vi "Cal BC (VIRef).vi"(8 "error in (no error)":errorcluster, 10 "BC in":variant, 11 "Domain_Evolut_1D in":refnum<class "NI_Domain_Evolut_1D.lvclass">) -> (0 "error out":errorcluster, 2 "BC out":variant, 3 "Domain_Evolut_1D out":refnum<class "NI_Domain_Evolut_1D.lvclass">)   [LabVIEW 2017, in "NI_PDE.lvlib" / "NI_Domain_Evolut_1D.lvclass"]
uses:
  <vilib>/gmath/pde.llb/DomainClass/Domain_Evolut_1D/NI_Domain_Evolut_1D.lvclass
  <vilib>/gmath/pde.llb/BCClass/BC_Evolut_1D_Numeric/BC Data.ctl
  <vilib>/gmath/pde.llb/Common/PDE_BC Type.ctl
  <vilib>/gmath/pde.llb/Common/PDE_BC Position 1D.ctl
  <vilib>/gmath/pde.llb/BCClass/BC_Evolut_1D_VIRef/BC Data.ctl
  <vilib>/gmath/pde.llb/DomainClass/Domain_Evolut_1D/NI_Domain_Evolut_1D.lvclass/NI_Domain_Evolut_1D.ctl
  <vilib>/Analysis/1siggen.llb/Ramp Pattern by Samples.vi
  <vilib>/gmath/NI_PDE.lvlib
  <vilib>/gmath/pde.llb/BCClass/BC_Evolut_1D_Numeric/NI_BC_Evolut_1D_Numeric.lvclass
  <vilib>/gmath/pde.llb/BCClass/BC_Evolut_1D_VIRef/NI_BC_Evolut_1D_VIRef.lvclass
  <vilib>/Analysis/NI_AALBase.lvlib
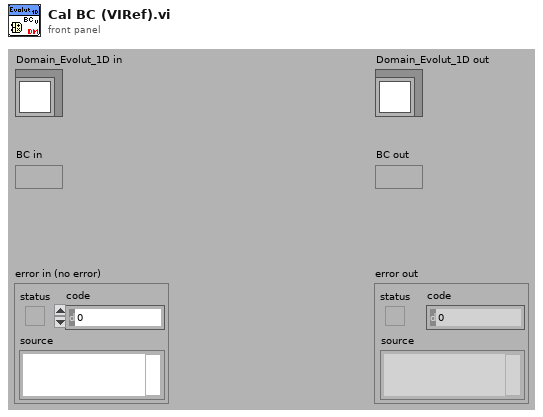
[diagram p1: front panel]
types:
  T1 = typedef "NI_PDE.lvlib/NI_BC_Evolut_1D_VIRef.lvclass/BC Data.ctl" = cluster{"type":T2, "position":T3, "G":refnum<vi>, "data":variant}
  T2 = typedef "NI_PDE.lvlib/PDE_BC Type.ctl" = i32
  T3 = typedef "NI_PDE.lvlib/PDE_BC Position 1D.ctl" = i32
  T4 = typedef "NI_PDE.lvlib/NI_BC_Evolut_1D_Numeric.lvclass/BC Data.ctl" = cluster{"type":T2, "position":T3, "G":dbl[]}
  T5 = cluster{"initial t":dbl, "final t":dbl, "# of t-points":i32}
  T6 = cluster{"start x":dbl, "end x":dbl, "# of x-points":i32}
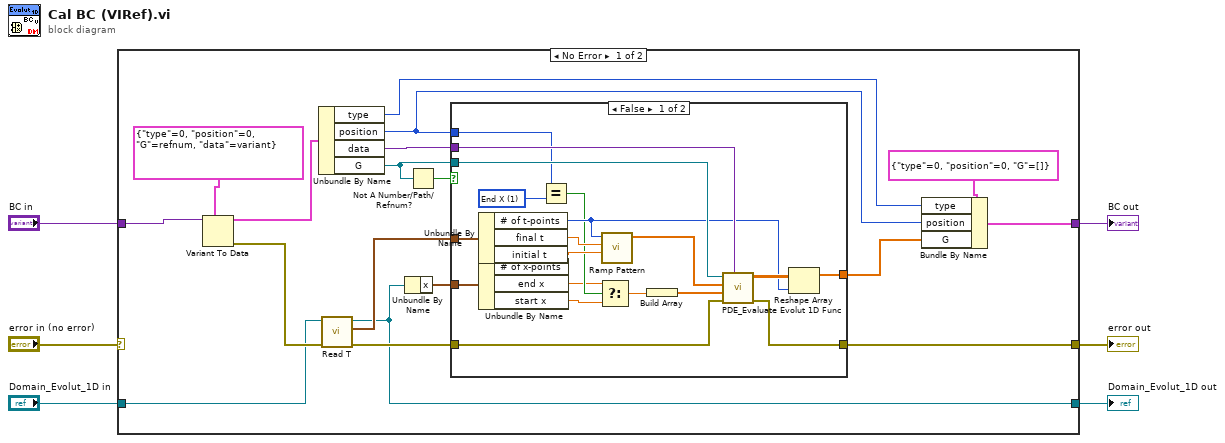
[diagram p0: block diagram]
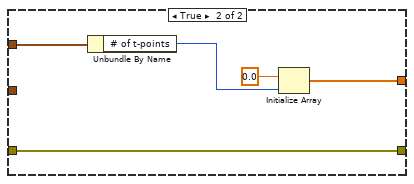
[diagram p2: hidden frame]
diagram:
  n1 = case shown="No Error" "error in (no error)" {
    selector: "error in (no error)" -> [_ w51]
    tunnel: "Domain_Evolut_1D in" -> [w10 w50]
    tunnel: [w7 w50] -> w6
    tunnel: [w13 w51] -> w5
    tunnel: [w14 w49] -> w2
    tunnel: "BC in" -> [w15 w49]
    frame No Error {
      n2 = Variant To Data(type=T1 {"type"=0, "position"=0, "G"=refnum, "data"=variant} ("BC data"), Variant=w15) -> (data=w21:T1, error out=w12:errorcluster)  [unwired: 1 in]
      n3 = Unbundle By Name(w21) -> ("type"=w23:T2, "position"=w24:T3, "data"=w18:variant, "G"=w17:refnum<vi>)
      n4 = call-dynamic "Read T.vi"("error in (no error)"=w12, "Domain_Evolut.lvclass in"=w10) -> ("error out"=w8:errorcluster, "t"=w11:T5, "Domain_Evolut.lvclass out"=w7:refnum<class "NI_Domain_Evolut_1D.lvclass">)  [unwired: 7 out]
      n5 = Unbundle By Name(w7) -> ("x"=w9:T6)
      n6 = Not A Number/Path/Refnum?(number/path/refnum=w17) -> (NaN/Path/Refnum?=w16:bool)
      n7 = case shown="False" w16 {
        tunnel: [w38 w48] -> w22
        tunnel: w11 -> [w43 w47]
        tunnel: w8 -> [w36 w45]
        tunnel: [w42 w45] -> w13
        tunnel: w17 -> [w41 _]
        tunnel: w18 -> [w40 _]
        tunnel: w9 -> [w35 _]
        tunnel: w24 -> [w25 _]
        frame False {
          w34 = T3 1 items=["Start X", "End X"] ("y")
          n8 = Unbundle By Name(w43) -> ("# of t-points"=w37:i32, "final t"=w32:dbl, "initial t"=w33:dbl)
          n9 = Unbundle By Name(w35) -> ("end x"=w30:dbl, "start x"=w29:dbl)  [unwired: 1 out]
          n10 = Equal?(x=w25, y=w34) -> (x = y?=w31:bool)
          n11 = Select(t=w30, s=w31, f=w29) -> (s? t:f=w28:dbl)
          n12 = call-poly <vilib>:"Ramp Pattern.vi"("start"=w33, "end"=w32, "samples"=w37) -> ("Ramp Pattern"=w27:dbl[])  [unwired: 7 in, 1 out]
          n13 = Build Array(w28) -> (w26:dbl[])
          n14 = call <vilib>:"PDE_Evaluate Evolut 1D Func.vi"("data"=w40, "error in (no error)"=w36, "X"=w26, "T"=w27, "VIRef"=w41) -> ("error out"=w42:errorcluster, "F(t, x)"=w39:dbl[][])  [unwired: 5 out]
          n15 = Reshape Array(w39, w37) -> (w38:dbl[])
        }
        frame True {
          n16 = Unbundle By Name(w47) -> ("# of t-points"=w44:i32)
          n17 = Initialize Array(0.0 ("element"), w44) -> (w48:dbl[])
        }
      }
      n18 = Bundle By Name(cluster=T4 {"type"=0, "position"=0, "G"=[]} ("BC data"), "type"=w23, "position"=w24, "G"=w22) -> (w14:T4)
    }
    frame Error {
    }
  }
  "Domain_Evolut_1D out" <- w6
  "error out" <- w5
  "BC out" <- w2
